vi "X in Y (Path Array)__jki_lib_array -- VI Tester.vi"(1 "array":path[](array[path]), 2 "element":path[](array[path])) -> (6 "element in array?":bool[](array[boolean]))   [LabVIEW 2013]
panel:
  # "Copyright © 2008 JKI. All rights reserved.\n\nAuthor: Jim Kring [jim.kring@jameskring.com]\n\nThis library is provided \"AS IS\" ,WITHOUT WARRANTIES OR \nCONDITIONS OF ANY KIND, either express or implied.\n\nJKI -- http://www.jameskring.com"
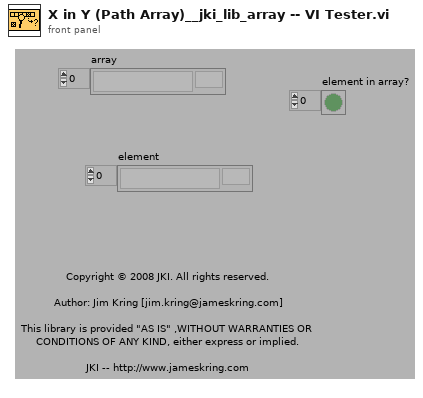
[diagram p1: front panel]
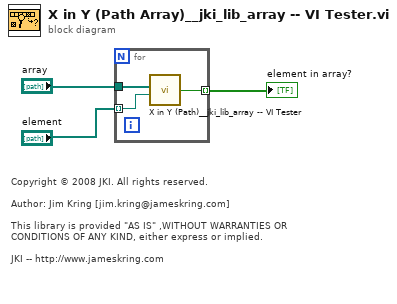
[diagram p0: block diagram]
diagram:
  # "Copyright © 2008 JKI. All rights reserved.\n\nAuthor: Jim Kring [jim.kring@jameskring.com]\n\nThis library is provided \"AS IS\" ,WITHOUT WARRANTIES OR \nCONDITIONS OF ANY KIND, either express or implied.\n\nJKI -- http://www.jameskring.com"
  n1 = for {
    tunnel: "array" -> [w6]
    tunnel: "element" -> [w5] mode=indexing
    tunnel: [w4] -> w1 mode=indexing
    n2 = call "X in Y (Path)__jki_lib_array -- VI Tester.vi"("array"=w6, "element"=w5) -> ("element in array?"=w4:bool)  [unwired: 5 in]
  }
  "element in array?" <- w1
